vi "Init value popup.vi"(8 "error in (no error)":errorcluster, 9 "Popup window reference":refnum<vi>, 10 "Bounds":T1, 11 "Control reference size override (none)":refnum<vi>) -> (0 "error out":errorcluster, 1 "Popup window reference out":refnum<vi>)   [LabVIEW 2018, in "D Datagrid Library.lvlib" / "DatagridElement.lvclass"]
doc: "Sets the caller VI's panel size to be the same size as the referenced control and moves the scroll position to the origin."
uses:
  DatagridElement.lvclass
  <vilib>/Utility/miscctls.llb/LVRectTypeDef.ctl
  <vilib>/Utility/miscctls.llb/LVPointTypeDef.ctl
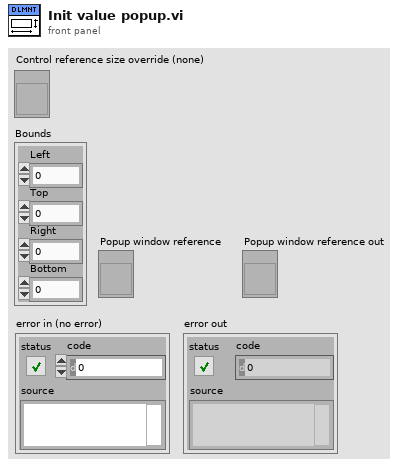
[diagram p1: front panel]
types:
  T1 = typedef "LVRectTypeDef.ctl" = cluster{"Left":i16, "Top":i16, "Right":i16, "Bottom":i16}
  T2 = enum32{"Invalid", "Standard", "Closed", "Hidden", "Minimized", "Maximized"}
  T3 = typedef "LVPointTypeDef.ctl" = cluster{"Horizontal":i16, "Vertical":i16}
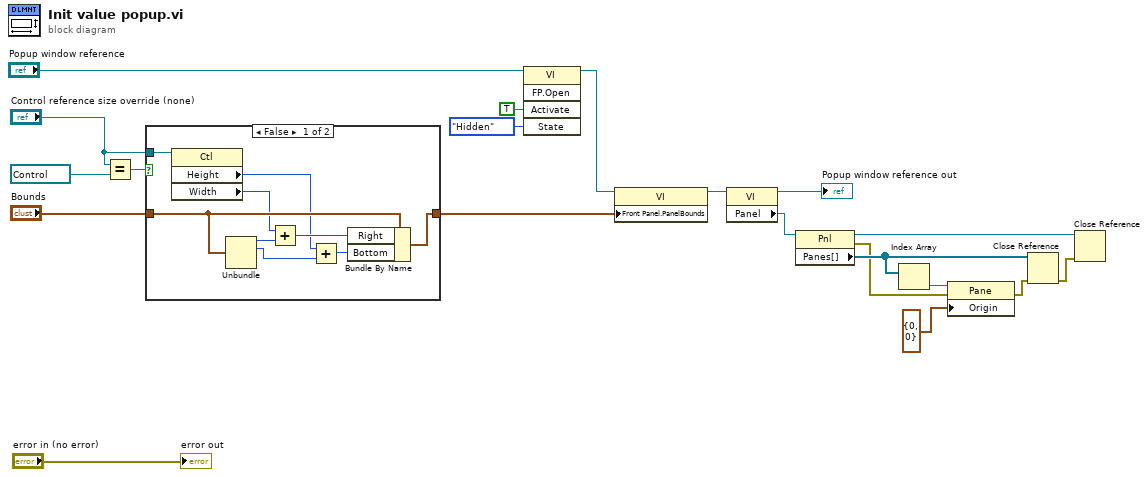
[diagram p0: block diagram]
diagram:
  n1 = Equal?(x="Control reference size override (none)", y=refnum<vi> refnum ("Control reference size override (none)")) -> (x = y?=w9:bool)
  n2 = case shown="False" w9 {
    tunnel: "Bounds" -> [w28 w30]
    tunnel: [w27 w30] -> w1
    tunnel: "Control reference size override (none)" -> [w29 _]
    frame False {
      n3 = property class="Ctl"(reference=w29) -> ("Height"=w21:u32, "Width"=w25:u32)  [unwired: 1 in, 2 out]
      n4 = Unbundle(w28) -> ("Left"=w26:i16, "Top"=w23:i16)  [unwired: 2 out]
      n5 = Add(x=w25, y=w26) -> (x+y=w24:u32)
      n6 = Add(x=w21, y=w23) -> (x+y=w22:u32)
      n7 = Bundle By Name(cluster=w28, "Right"=w24, "Bottom"=w22) -> (w27:T1)
    }
    frame True {
    }
  }
  n8 = invoke class="VI" method="FP.Open"(reference="Popup window reference", "Activate"=TRUE ("Activate?"), "State"=T2."Hidden") -> (reference out=w4:refnum<vi>)  [unwired: 2 in, 4 out]
  n9 = property class="VI"(reference=w4, "Front Panel.PanelBounds"=w1) -> (reference out=w11:refnum<vi>)  [unwired: 1 in, 1 out]
  n10 = property class="VI"(reference=w11) -> (reference out=→"Popup window reference out":refnum<vi>, "Panel"=w12:refnum<vi>)  [unwired: 1 in, 1 out]
  n11 = property class="Pnl"(reference=w12) -> (reference out=w16:refnum<vi>, error out=w15:errorcluster, "Panes[]"=w19:refnum<vi>[])  [unwired: 1 in]
  n12 = Index Array(array=w19) -> (element=w13:refnum<vi>)  [unwired: 1 in]
  n13 = property class="Pane"(reference=w13, error in=w15, "Origin"=T3 {"Horizontal"=0, "Vertical"=0}) -> (error out=w17:errorcluster)  [unwired: 1 out]
  n14 = Close Reference(reference=w19, error in (no error)=w17) -> (error out=w18:errorcluster)
  n15 = Close Reference(reference=w16, error in (no error)=w18) -> ()  [unwired: 1 out]
  "error out" <- "error in (no error)"
